vi "string_prepare(SubVI).vi"(11 "read string":string) -> (3 "String":string)   [LabVIEW 2017]
doc: "SubVI to initially prepare string read from car."
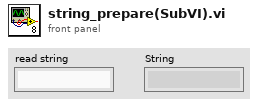
[diagram p1: front panel]
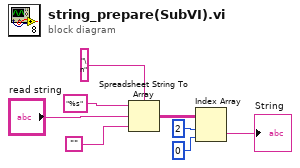
[diagram p0: block diagram]
diagram:
  n1 = Spreadsheet String To Array(delimiter (Tab)="\n", format string="%s" ("spreadsheet string"), spreadsheet string="read string", array type (2D Dbl)="") -> (array=w5:string[][])
  n2 = Index Array(array=w5, index (row)=2, index (col)=0 ("disabled index (col)")) -> (element=→"String":string)
